vi "Trav_single_profile.vi"(3 "Simulate/Run":T1, 5 "Traverse line":T2 {"Row Duration (mins)" format="%#.1f"; "Row No" min=0; "Trace Gas Concentration (%)" min=0.0 format="%#.2f"; "Emission Rate (l/min)" format="%#.2f"; "Tunnel Speed" format="%#.2f"; "Start X" format="%#.2f"; "Start Y" format="%#.2f"; "Start Z" format="%#.2f"; "End X" format="%#.2f"; "End Y" format="%#.2f"; "End Z" format="%#.2f"; "Averaging time (min)" min=0.0 format="%#.1f"}) -> (0 "Error Messages":string, 1 "Status":T5, 2 "Traverse line Out":T2 {"Row Duration (mins)" format="%#.1f"; "Row No" min=0; "Trace Gas Concentration (%)" min=0.0 format="%#.2f"; "Emission Rate (l/min)" format="%#.2f"; "Tunnel Speed" format="%#.2f"; "Start X" format="%#.2f"; "Start Y" format="%#.2f"; "Start Z" format="%#.2f"; "End X" format="%#.2f"; "End Y" format="%#.2f"; "End Z" format="%#.2f"; "Averaging time (min)" min=0.0 format="%#.1f"})   [LabVIEW 2010]
uses:
  Gen Trav/Multi_Run_Status.ctl
  Gen Trav/Traverse_cluster.ctl
  Gen Trav/Spacing.ctl
  Controls/Multi_run_mode.ctl
  Controls/User_Specific_mode.ctl
  Controls/Save_Data.ctl
  Controls/Setup.ctl
  ADAM Client/Sub VIs/ADAM Controls/Traverse_Level_State.ctl
  Controls/Overhead.ctl
  Globals/Trav_pos_global.vi
  Globals/Meas_global.vi
panel:
  out "Pause message":string
  in  "Pause":bool
  out "Current position":dbl[](array[numeric]) format="%.2f"
  in  "stop":bool
  in  "Array of Positions":dbl[][](array[numeric]) format="%.2f"
  out "Abcissa copy":string="Y (mm)"
  out "Abcissa":string="Y (mm)"
  in  "Plot 1":i32[](listbox)=[1]
  out "Started Profile at:":string="16/9/98 12:33"
  out "Currently on point":i32=9
  out "U":cluster{dbl[], dbl[]}[](graph)
  out "% u'/U":cluster{dbl[], dbl[]}[](graph)
  # "X           Y            Z"
  # "Start"
  # "End"
  # "X           Y            Z"
  # "Start"
  # "End"
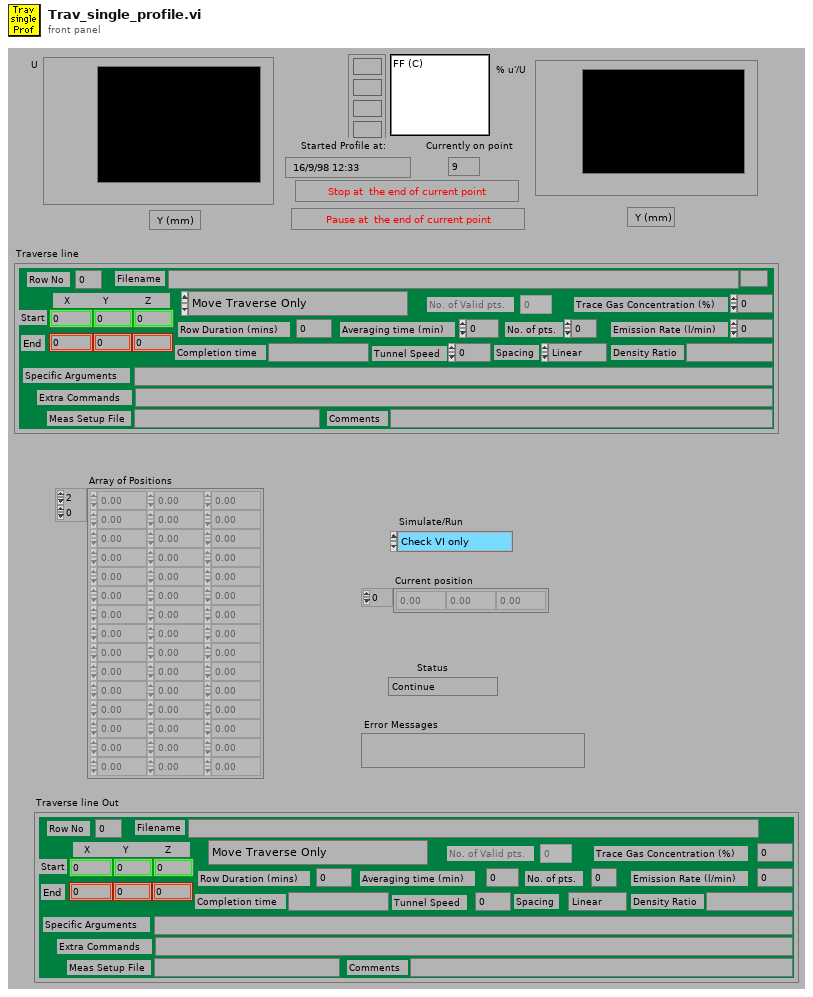
[diagram p1: front panel]
types:
  T1 = typedef "User_Specific_mode.ctl" = enum16{"Check VI only", "Run VI"}
  T2 = typedef "Traverse_cluster.ctl" = cluster{"Start X":dbl, "Start Y":dbl, "Start Z":dbl, "End X":dbl, "End Y":dbl, "End Z":dbl, "No. of pts.":i32, "Spacing":T3, "Filename":path, "Tunnel Speed":dbl, "Averaging time (min)":dbl, "Extra Commands":string, "Specific Arguments":string, "Emission Rate (l/min)":dbl, "Trace Gas Concentration (%)":dbl, "Density Ratio":string, "Comments":string, "Row No":i32, "Row Type Selector":T4, "Completion time":string, "Row Duration (mins)":dbl, "No. of Valid pts.":i32, "Meas Setup File":string}
  T3 = typedef "Spacing.ctl" = enum16{"Linear", "Log", "Gauss", "Specified", "N/A"}
  T4 = typedef "Multi_run_mode.ctl" = enum16{"Move Traverse Only", "Set Tunnel Speed Only", "Set Source Only", "Set Measurement Conditions", "Single Measurement", "Vertical Profile", "Lateral Profile", "Longitudinal Profile", "Explore Volume", "Multi-Axis Profile", "Auto Calibrate", "Meas Fast FID Bkgnd", "Check Beam Power", "Scanning Valve Measurement", "Run VI Named:", "Set ADAM Ch", "Wait (minutes)", "Send Message", "Synchronize With:", "Fall Back to this Row", "Turn Off Row Repeating", "Blank Row"}
  T5 = typedef "Multi_Run_Status.ctl" = enum16{"Continue", "Jump to Next Point", "Jump to Next Row", "Jump To Fall Back", "Terminate Run"}
  T6 = typedef "Save_Data.ctl" = enum16{"Save No Data", "Save Data"}
  T7 = typedef "Setup.ctl" = enum16{"Run Program", "Show Setup", "Save Current Setup", "Setup Front Panel"}
  T8 = typedef "Traverse_Level_State.ctl" = enum16{"Running", "Complete"}
  T9 = typedef "Overhead.ctl" = enum16{"Update total times", "Read Current Overhead", "Re Scale totals to 3 hrs", "Initialise totals to 3hr"}
  T10 = typedef "Status_Cluster.ctl" = cluster{"Status":T5, "Error Type":string, "Error Description":string}
  T11 = typedef "Velocity_cluster.ctl" = cluster{"Name":string, "U":dbl, "u^2":dbl, "u^3/(u^2)^(1.5)":dbl, "u^4/(u^2)^2 -3":dbl, "% u'/U":dbl, "Mean % Err":dbl, "u^4":dbl}
  T12 = typedef "Analysis_type_cluster.ctl" = cluster{"Analysis type":T13, "Indicies":i32[], "Name":string, "Inst Array":T14, "Info index":i32}
  T13 = typedef "Analysis_type_Enum.ctl" = enum16{"Slow Response", "Fast Response", "Weighted Fast Response", "Fast FID", "Weighted Fast FID", "Cross Wire", "Weighted Cross Wire", "Weighted LDA"}
  T14 = typedef "Instrument_Array.ctl" = enum16{"PWA", "LDA", "Analogue"}
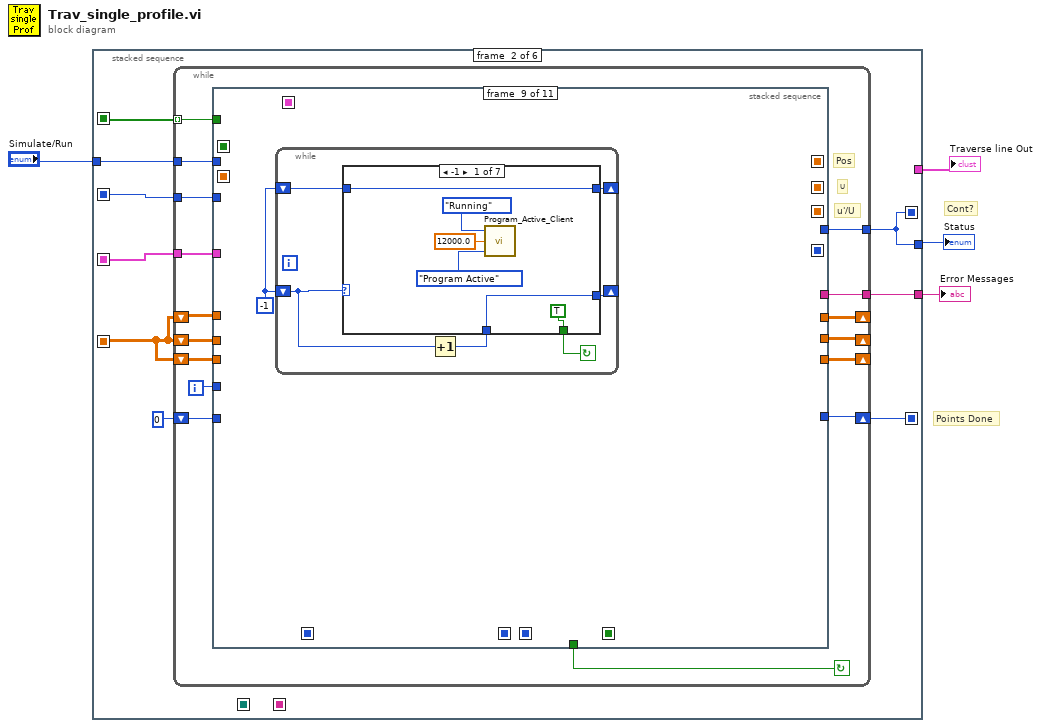
[diagram p0: block diagram]
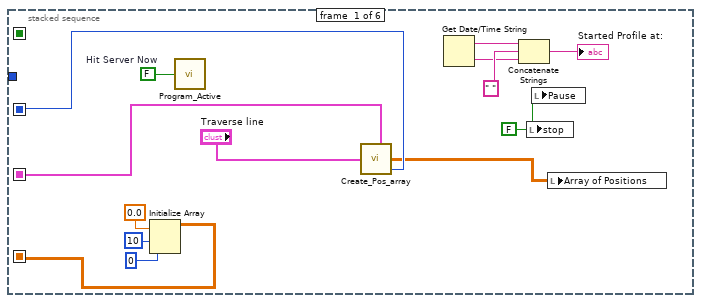
[diagram p2: hidden frame]
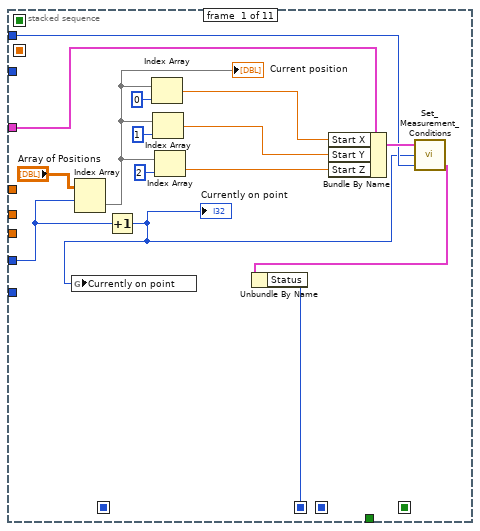
[diagram p3: hidden frame]
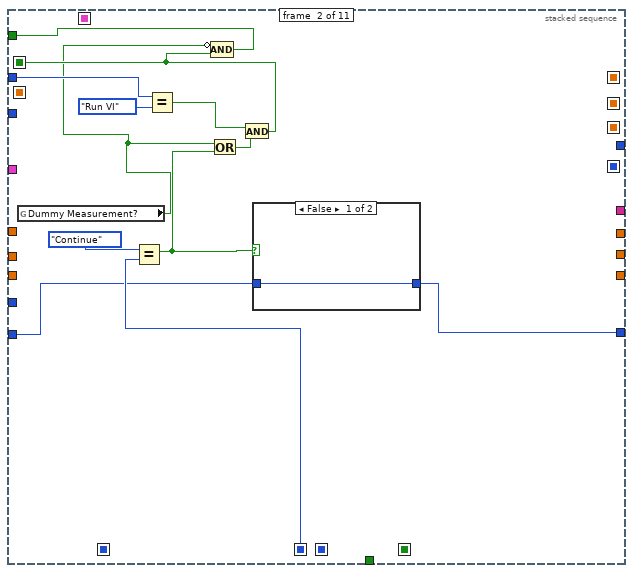
[diagram p4: hidden frame]
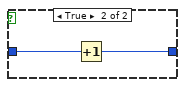
[diagram p5: hidden frame]
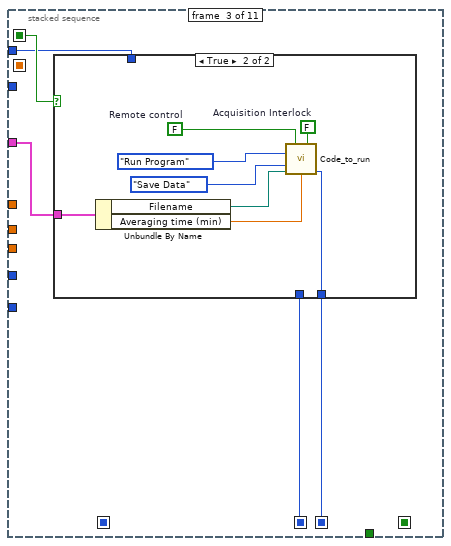
[diagram p6: hidden frame]
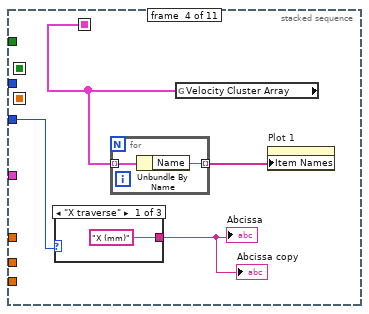
[diagram p8: hidden frame]
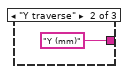
[diagram p9: hidden frame]
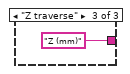
[diagram p10: hidden frame]
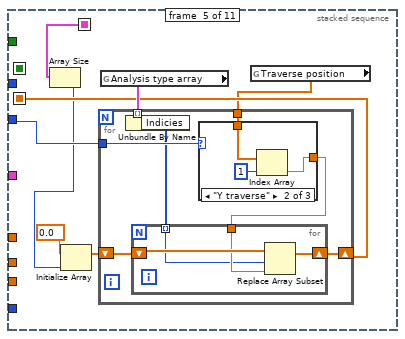
[diagram p11: hidden frame]
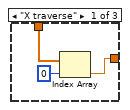
[diagram p12: hidden frame]
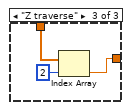
[diagram p13: hidden frame]
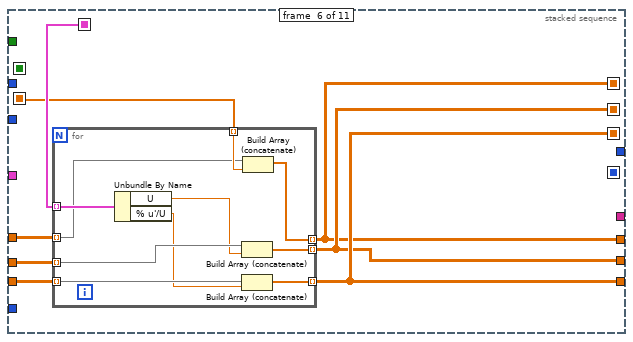
[diagram p14: hidden frame]
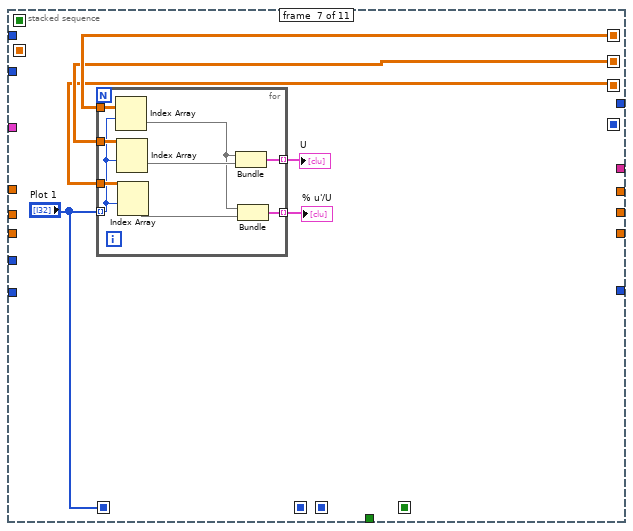
[diagram p15: hidden frame]
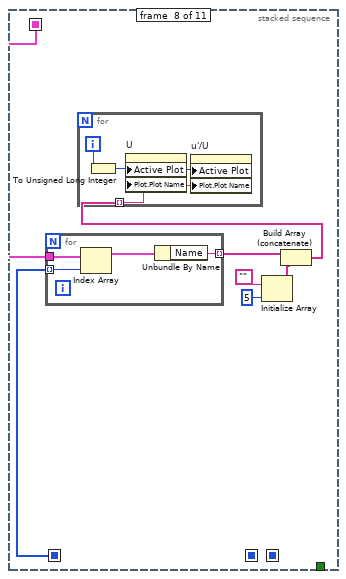
[diagram p16: hidden frame]
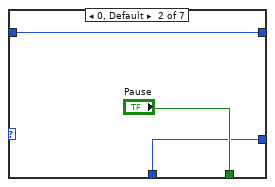
[diagram p17: hidden frame]
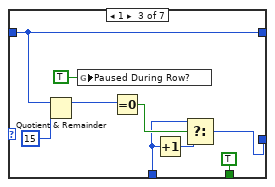
[diagram p18: hidden frame]
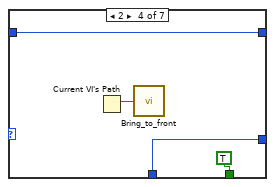
[diagram p19: hidden frame]
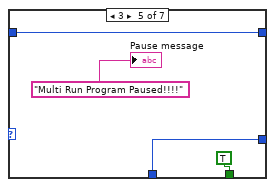
[diagram p20: hidden frame]
diagram:
  # "Points Done"
  # "Cont?"
  n1 = stacked-sequence {
    seq-local: [w11 _ _ _ _ _] -> [_ w26 _ _ _ _]
    seq-local: [w10 _ _ _ _ _] -> [_ w27 _ _ _ _]
    seq-local: [_ _ w276 _ _ _] -> [_ _ _ _ w300 _]
    seq-local: [_ _ _ w283 _ _] -> [_ _ _ _ w299 _]
    seq-local: [_ w25 _ _ _ _] -> [_ _ _ _ _ _]
    seq-local: [_ w23 _ _ _ _] -> [_ _ _ w280 w298 _]
    seq-local: [_ w21 _ _ _ _] -> [_ _ _ _ _ w305]
    seq-local: [w6 _ _ _ _ _] -> [_ w20 _ _ _ w307]
    tunnel: [_ w25 _ _ _ _] -> w2
    tunnel: [_ _ _ _ _ w317] -> w4
    tunnel: "Simulate/Run" -> [_ w24 _ _ _ w316]
    tunnel: [_ w19 _ _ _ _] -> w1
    frame #0 {
      w8 = FALSE ("stop")
      w9 = FALSE  # Hit Server Now
      n2 = Initialize Array(0.0, 10, 0) -> (w11:dbl[][])
      n3 = call "Program_Active.vi"("Hit Server Now"=w9) -> ()
      n4 = call "Create_Pos_array.vi"("Traverse line"="Traverse line") -> ("Traverse line Out"=w6:T2, "Array of Positions"=w5:dbl[][], "Axis Traversed"=w10:enum16{"X traverse", "Y traverse", "Z traverse"})  [unwired: 5 in, 1 out]
      n5 = Get Date/Time String() -> (date string=w17:string, time string=w16:string)  [unwired: 3 out]
      n6 = Concatenate Strings(w17, " ", w16) -> (→"Started Profile at:":string)
      n7 = local write "stop"(w8) -> ()
      n8 = local write "Pause"(w8) -> ()
      n9 = local write "Array of Positions"(w5) -> ()
    }
    frame #1 {
      n10 = while {
        shift-left: 0 -> [w30]
        shift-right: [w29] -> w21
        tunnel: [w31] -> w23 mode=indexing
        tunnel: w20 -> [w32]
        tunnel: w24 -> [w33]
        tunnel: [w34] -> w25
        shift-left: w26 -> [w37]
        shift-right: [w36] -> _
        tunnel: w27 -> [w38]
        shift-left: w26 -> [w40]
        shift-right: [w39] -> _
        shift-left: w26 -> [w42]
        shift-right: [w41] -> _
        tunnel: [w28] -> w19
        i -> [w43]
        stop <- w35 continue-if-true
        # "Pos"
        # "U"
        # "u'/U"
        n11 = stacked-sequence {
          seq-local: [_ _ _ _ w102 _ _ _ _ _ _] -> [_ _ _ _ _ w127 _ _ _ _ _]
          seq-local: [_ _ _ w91 _ _ _ _ _ _ _] -> [_ _ _ _ w101 w130 _ w158 _ _ _]
          seq-local: [_ _ _ _ _ w125 _ _ _ _ _] -> [_ _ _ _ _ _ w148 _ _ _ _]
          seq-local: [_ _ _ _ _ w128 _ _ _ _ _] -> [_ _ _ _ _ _ w147 _ _ _ _]
          seq-local: [_ _ _ _ _ w129 _ _ _ _ _] -> [_ _ _ _ _ _ w146 _ _ _ _]
          seq-local: [_ _ _ _ _ _ "Plot 1" _ _ _ _] -> [_ _ _ _ _ _ _ w164 _ _ _]
          seq-local: [_ _ w77 _ _ _ _ _ _ _ _] -> [_ _ _ _ _ _ _ _ _ w222 _]
          seq-local: [w48 _ _ _ _ _ _ _ _ _ _] -> [_ w68 w75 _ _ _ _ _ _ _ _]
          seq-local: [_ w61 _ _ _ _ _ _ _ _ _] -> [_ _ w76 _ _ _ _ _ _ _ _]
          seq-local: [_ _ _ _ _ _ _ _ _ w217 _] -> [_ _ _ _ _ _ _ _ _ _ w238]
          seq-local: [_ _ _ _ _ _ _ _ _ w216 _] -> [_ _ _ _ _ _ _ _ _ _ w232]
          tunnel: w43 -> [w45 _ _ _ _ _ _ _ _ w228 w235]
          tunnel: w42 -> [_ _ _ _ _ w132 _ _ _ _ _]
          tunnel: [_ _ _ _ _ w128 _ _ _ _ _] -> w41
          tunnel: w40 -> [_ _ _ _ _ w131 _ _ _ _ _]
          tunnel: [_ _ _ _ _ w129 _ _ _ _ _] -> w39
          tunnel: w38 -> [_ _ _ w89 w103 _ _ _ _ _ _]
          tunnel: w37 -> [_ _ _ _ _ w126 _ _ _ _ _]
          tunnel: [_ _ _ _ _ w125 _ _ _ _ _] -> w36
          tunnel: [_ _ _ _ _ _ _ _ _ w217 _] -> w35
          tunnel: w32 -> [w52 _ w78 _ _ _ _ _ _ _ w236]
          tunnel: [_ _ _ _ _ _ _ _ _ _ w234] -> w34
          tunnel: w33 -> [w50 w70 w74 _ _ _ _ _ _ _ w237]
          tunnel: [_ w60 _ _ _ _ _ _ _ _ _] -> w31
          tunnel: w30 -> [_ w65 _ _ _ _ _ _ _ _ _]
          tunnel: [_ w64 _ _ _ _ _ _ _ _ _] -> w29
          tunnel: [_ _ _ _ _ _ _ _ _ _ w233] -> w28
          frame #0 {
            n12 = Index Array(array="Array of Positions", index (row)=w45) -> (element=w44:dbl[])  [unwired: 1 in]
            "Current position" <- w44
            n13 = Increment(x=w45) -> (x+1=w47:i32)
            "Currently on point" <- w47
            n14 = global write "Trav_pos_global.vi" "Currently on point"(w47) -> ()
            n15 = Index Array(array=w44, index=0 ("Index")) -> (element=w55:dbl)
            n16 = Index Array(array=w44, index=1 ("Index")) -> (element=w54:dbl)
            n17 = Index Array(array=w44, index=2 ("Index")) -> (element=w53:dbl)
            n18 = Bundle By Name(cluster=w52, "Start X"=w55, "Start Y"=w54, "Start Z"=w53) -> (w51:T2)
            n19 = call "Set_Measurement_Conditions.vi"("Simulate/Run"=w50, "Currently on Point"=w47, "Traverse line"=w51) -> ("Status Cluster"=w49:T10)  [unwired: 2 out]
            n20 = Unbundle By Name(w49) -> ("Status"=w48:T5)
          }
          frame #1 {
            n21 = global read "Trav_pos_global.vi" "Dummy Measurement?"() -> (w59:bool)
            n22 = Equal?(x=Multi_Run_Status."Continue" ("Status"), y=w68) -> (x = y?=w63:bool)
            n23 = Equal?(x=w70, y=User_Specific_mode."Run VI" ("Simulate/Run")) -> (x = y?=w66:bool)
            n24 = Or(x=w59, y=w63) -> (x .or. y?=w62:bool)
            n25 = And(x=w66, y=w62) -> (x .and. y?=w61:bool)
            n26 = Compound Arithmetic op=AND(invert w59, w61) -> (w60:bool)
            n27 = case shown="False" w63 {
              tunnel: w65 -> [w71 w73]
              tunnel: [w71 w72] -> w64
              frame False {
              }
              frame True {
                n28 = Increment(x=w73) -> (x+1=w72:i32)
              }
            }
          }
          frame #2 {
            n29 = case shown="True" w76 {
              tunnel: w78 -> [_ w87]
              tunnel: [w79 w86] -> w77
              tunnel: w75 -> [w79 _]
              tunnel: w74 -> [_ _]
              frame False {
              }
              frame True {
                w82 = FALSE  # Acquisition Interlock
                w85 = FALSE  # Remote control
                n30 = Unbundle By Name(w87) -> ("Filename"=w83:path, "Averaging time (min)"=w84:dbl)
                n31 = call "Code_to_run.vi"("Acquisition Interlock"=w82, "setup"=Setup."Run Program", "Remote control"=w85, "File"=Save_Data."Save Data", "Results Filename"=w83, "Averaging time (min)"=w84) -> ("Status"=w86:T5)  [unwired: 5 in, 4 out]
              }
            }
          }
          frame #3 {
            n32 = case shown="\"X traverse\"" w89 {
              tunnel: ["X (mm)" "Y (mm)" "Z (mm)"] -> w88
              frame "X traverse" {
              }
              frame "Y traverse" {
              }
              frame "Z traverse" {
              }
            }
            "Abcissa" <- w88
            "Abcissa copy" <- w88
            n33 = global read "Meas_global.vi" "Velocity Cluster Array"() -> (w91:T11[])
            n34 = for {
              tunnel: w91 -> [w96] mode=indexing
              tunnel: [w95] -> w90 mode=indexing
              n35 = Unbundle By Name(w96) -> ("Name"=w95:string)
            }
            n36 = property on="Plot 1" class="LstBox (strict)"("Item Names"=w90) -> ()  [unwired: 2 in, 2 out]
          }
          frame #4 {
            n37 = Array Size(array=w101) -> (size(s)=w100:i32)
            n38 = Initialize Array(0.0, w100) -> (w98:dbl[])
            n39 = global read "Meas_global.vi" "Analysis type array"() -> (w104:T12[])
            n40 = global read "Trav_pos_global.vi" "Traverse position"() -> (w97:dbl[])
            n41 = for {
              shift-right: [w108] -> w102
              shift-left: w98 -> [w109]
              tunnel: w104 -> [w111] mode=indexing
              tunnel: w103 -> [w110]
              tunnel: w97 -> [w105]
              n42 = Unbundle By Name(w111) -> ("Indicies"=w106:i32[])
              n43 = case shown="\"Y traverse\"" w110 {
                tunnel: [w117 w120 w122] -> w107
                tunnel: w105 -> [w118 w119 w123]
                frame "X traverse" {
                  n44 = Index Array(array=w118, index=0) -> (element=w117:dbl)
                }
                frame "Y traverse" {
                  n45 = Index Array(array=w119, index=1) -> (element=w120:dbl)
                }
                frame "Z traverse" {
                  n46 = Index Array(array=w123, index=2) -> (element=w122:dbl)
                }
              }
              n47 = for {
                shift-right: [w114] -> w108
                shift-left: w109 -> [w115]
                tunnel: w107 -> [w113]
                tunnel: w106 -> [w112] mode=indexing
                n48 = Replace Array Subset(array=w115, new element=w113, index=w112) -> (w114:dbl[])
              }
            }
          }
          frame #5 {
            n49 = for {
              tunnel: w132 -> [w142] mode=indexing
              tunnel: [w140] -> w128 mode=indexing
              tunnel: w131 -> [w139] mode=indexing
              tunnel: [w137] -> w129 mode=indexing
              tunnel: w130 -> [w136] mode=indexing
              tunnel: w127 -> [w135] mode=indexing
              tunnel: w126 -> [w134] mode=indexing
              tunnel: [w133] -> w125 mode=indexing
              n50 = Unbundle By Name(w136) -> ("U"=w141:dbl, "% u'/U"=w138:dbl)
              n51 = Build Array (concatenate)(w142, w141) -> (w140:dbl[])
              n52 = Build Array (concatenate)(w139, w138) -> (w137:dbl[])
              n53 = Build Array (concatenate)(w134, w135) -> (w133:dbl[])
            }
          }
          frame #6 {
            n54 = for {
              tunnel: "Plot 1" -> [w149] mode=indexing
              tunnel: w148 -> [w157]
              tunnel: w147 -> [w156]
              tunnel: w146 -> [w155]
              tunnel: [w151] -> w145 mode=indexing
              tunnel: [w150] -> w144 mode=indexing
              n55 = Index Array(array=w157, index (row)=w149) -> (element=w153:dbl[])  [unwired: 1 in]
              n56 = Index Array(array=w156, index (row)=w149) -> (element=w154:dbl[])  [unwired: 1 in]
              n57 = Index Array(array=w155, index (row)=w149) -> (element=w152:dbl[])  [unwired: 1 in]
              n58 = Bundle(w153, w154) -> (w150:cluster{dbl[], dbl[]})  [unwired: 1 out]
              n59 = Bundle(w153, w152) -> (w151:cluster{dbl[], dbl[]})  [unwired: 1 out]
            }
            "U" <- w144
            "% u'/U" <- w145
          }
          frame #7 {
            n60 = for {
              tunnel: w164 -> [w168] mode=indexing
              tunnel: w158 -> [w166]
              tunnel: [w165] -> w161 mode=indexing
              n61 = Index Array(array=w166, index=w168) -> (element=w167:T11)
              n62 = Unbundle By Name(w167) -> ("Name"=w165:string)
            }
            n63 = Initialize Array("", 5) -> (w160:string[])
            n64 = Build Array (concatenate)(w161, w160) -> (w159:string[])
            n65 = for {
              tunnel: w159 -> [w169] mode=indexing
              i -> [w171]
              n66 = To Unsigned Long Integer(number=w171) -> (unsigned 32bit integer=w170:u32)
              n67 = property on="U" class="XYGraph (strict)"("Active Plot"=w170, "Plot.Plot Name"=w169) -> ()  [unwired: 2 in, 2 out]
              n68 = property on="u'/U" class="XYGraph (strict)"("Active Plot"=w170, "Plot.Plot Name"=w169) -> ()  [unwired: 2 in, 2 out]
            }
          }
          frame #8 {
            w172 = -1
            n69 = while {
              shift-left: w172 -> [w173]
              shift-right: [w174] -> _
              shift-left: w172 -> [w177]
              shift-right: [w178] -> _
              stop <- w175 continue-if-true
              n70 = Increment(x=w177) -> (x+1=w176:i32)
              n71 = case shown="-1" w177 {
                tunnel: [w183 w186 w190 w200 w203 w207 0] -> w178
                tunnel: w176 -> [w183 w186 w192 w200 w203 w207 _]
                tunnel: [TRUE ("Pause") "Pause" TRUE ("Pause") TRUE ("Pause") TRUE ("Pause") TRUE ("Pause") TRUE ("Pause")] -> w175
                tunnel: [w182 w185 w188 w197 w201 w205 w210] -> w174
                tunnel: w173 -> [w182 w185 w188 w197 w201 w205 w211]
                frame -1 {
                  n72 = call "Program_Active_Client.vi"("Mode"=enum16{"Program Active", "Traverse Level State"}."Program Active", "Time till next contact (Sec)"=12000.0, "Traverse level State"=Traverse_Level_State."Running") -> ()  [unwired: 3 out]
                }
                frame 0, Default {
                }
                frame 1 {
                  n73 = Quotient & Remainder(x=w188, y=15) -> (x-y*floor(x/y)=w194:i32)  [unwired: 1 out]
                  n74 = global write "Trav_pos_global.vi" "Paused During Row?"(TRUE ("Paused During Row?")) -> ()
                  n75 = Equal To 0?(x=w194) -> (x = 0?=w193:bool)
                  n76 = Increment(x=w192) -> (x+1=w191:i32)
                  n77 = Select(t=w192, s=w193, f=w191) -> (s? t:f=w190:i32)
                }
                frame 2 {
                  n78 = Current VI's Path() -> (path=w198:path)
                  n79 = call "Bring_to_front.vi"("path"=w198) -> ()
                }
                frame 3 {
                  "Pause message" <- "Multi Run Program Paused!!!!" ("Pause message")
                }
                frame 4 {
                  n80 = property on="Pause message" class="Str"("Visible"=TRUE) -> ()  [unwired: 2 in, 2 out]
                  n81 = Wait Until Next ms Multiple(millisecond multiple=u32 1500) -> ()  [unwired: 1 out]
                }
                frame 5 {
                  n82 = Increment(x=w211) -> (x+1=w210:i32)
                  n83 = property on="Pause message" class="Str"("Visible"=FALSE) -> ()  [unwired: 2 in, 2 out]
                  n84 = Wait Until Next ms Multiple(millisecond multiple=u32 1500) -> ()  [unwired: 1 out]
                }
              }
            }
          }
          frame #9 {
            n85 = Increment(x=w228) -> (x+1=w227:i32)
            n86 = local read "Array of Positions"() -> (w218:dbl[][])
            n87 = case shown="\"Jump to Next Point\"" w222 {
              tunnel: [TRUE TRUE FALSE] -> w225
              frame "Continue" {
              }
              frame "Jump to Next Point" {
              }
              frame "Jump to Next Row", Default {
              }
            }
            n88 = Array Size(array=w218) -> (size(s)=w221:i32[])
            n89 = Index Array(array=w221, index=0 ("Index")) -> (element=w219:i32)
            n90 = Less?(x=w227, y=w219) -> (x < y?=w226:bool)
            n91 = Compound Arithmetic op=AND(w225, invert "stop", w226) -> (w217:bool)
            n92 = Select(t=Multi_Run_Status."Terminate Run" ("Status"), s="stop", f=w222) -> (s? t:f=w216:T5)
          }
          frame #10 {
            n93 = case shown="True" w238 {
              tunnel: w237 -> [_ w247]
              tunnel: w236 -> [_ w246]
              tunnel: w235 -> [_ w245]
              tunnel: [w240 w242] -> w234
              tunnel: ["" w241] -> w233
              tunnel: w232 -> [w240 _]
              frame False {
              }
              frame True {
                n94 = case shown="\"Check VI only\"" w247 {
                  tunnel: w246 -> [w263 _]
                  tunnel: w245 -> [w258 _]
                  tunnel: [w248 timestamp(0 s since 1904-01-01)] -> w244
                  frame "Check VI only" {
                    n95 = Increment(x=w258) -> (x+1=w256:i32)
                    n96 = Unbundle By Name(w263) -> ("Averaging time (min)"=w260:dbl)
                    n97 = global read "Trav_pos_global.vi" "Simulation Time"() -> (w250:timestamp)
                    n98 = To Double Precision Float(number=w250) -> (double precision float=w251:dbl)
                    n99 = Multiply(x=60.0, y=w260) -> (x*y=w259:dbl)
                    n100 = Add(x=w259, y=10.0 ("Scalable Time (Sec)")) -> (x+y=w257:dbl)
                    n101 = Multiply(x=w257, y=w256) -> (x*y=w254:dbl)
                    n102 = call "Overhead_Factor.vi"("Mode"=Overhead."Read Current Overhead") -> ("Current Overhead Factor"=w255:dbl)  [unwired: 3 in]
                    n103 = Multiply(x=w255, y=w254) -> (x*y=w252:dbl)
                    n104 = Add(x=w251, y=w252) -> (x+y=w249:dbl)
                    n105 = To Time Stamp(1:w249) -> (0:w248:timestamp)
                  }
                  frame "Run VI" {
                  }
                }
                n106 = call "Run_FFID_Bkgnd.vi"("Simulated Time"=w244, "Run Now?"=FALSE, "Simulate/Run"=w247) -> ("Error Messages"=w241:string, "Status"=w242:T5)  [unwired: 1 out]
              }
            }
          }
        }
      }
    }
    frame #2 {
      n107 = global read "Meas_global.vi" "Start Time of experiment"() -> (w266:dbl)
      n108 = global read "Meas_global.vi" "Raw data file"() -> (w278:path)
      n109 = Strip Path(path=w278) -> (stripped path=w277:path)  [unwired: 1 out]
      n110 = call "Sec_to_date_filename.vi"("seconds"=w266) -> ("Day"=w268:string, "Time"=w269:string)  [unwired: 2 out]
      n111 = Format Into String(format string="Cmd_%s_%s.xls", w268, w269) -> (resulting string=w271:string)  [unwired: 2 in, 1 out]
      n112 = call "Fast_string_Replace.vi"("Replace match with:"="-", "Input String"=w271, "regular expression"=":") -> ("Output String"=w274:string)  [unwired: 2 out]
      n113 = call "Fast_string_Replace.vi"("Replace match with:"="", "Input String"=w274, "regular expression"=" ") -> ("Output String"=w265:string)  [unwired: 2 out]
      n114 = Build Path(base path=w277, name or relative path=w265) -> (appended path=w276:path)
    }
    frame #3 {
      w289 = "\t"
      n115 = local read "Array of Positions"() -> (w282:dbl[][])
      n116 = Number To Fractional String(number=w282, precision (6)=i16 2) -> (F-format string=w281:string[][])  [unwired: 2 out]
      n117 = for {
        tunnel: w281 -> [w294] mode=indexing
        tunnel: w280 -> [w293] mode=indexing
        tunnel: [w291] -> w279 mode=indexing
        n118 = case shown="False" w293 {
          tunnel: ["Unobtainable Position" ""] -> w292
          frame False {
          }
          frame True {
          }
        }
        n119 = Build Array (concatenate)(w294, w292) -> (w291:string[])
      }
      n120 = Concatenate Strings("X", w289, "Y", w289, "Z") -> (w284:string)
      n121 = call "2D_array_to_string.vi"("2D data array"=w279, "Column titles  (separated by tabs)"=w284, "Array title"="Requested positions") -> ("Output string"=w283:string)
    }
    frame #4 {
      n122 = Or Array Elements(Boolean array=w298) -> (logical OR=w297:bool)
      n123 = case shown="True" w297 {
        tunnel: w300 -> [_ w303]
        tunnel: w299 -> [_ w301]
        frame False {
        }
        frame True {
          w302 = FALSE  # Lock File
          w304 = TRUE  # append to file? (new file:F)
          n124 = call "Write_Characters_To_File.vi"("file path (dialog if empty)"=w303, "character string"=w301, "append to file? (new file:F)"=w304, "Lock File"=w302) -> ()  [unwired: 1 in, 4 out]
        }
      }
    }
    frame #5 {
      n125 = local read "Array of Positions"() -> (w309:dbl[][])
      n126 = Array Size(array=w309) -> (size(s)=w311:i32[])
      n127 = Index Array(array=w311, index=0 ("Index")) -> (element=w308:i32)
      n128 = Bundle By Name(cluster=w307, "No. of Valid pts."=w305) -> (w306:T2)
      n129 = Not Equal?(x=w308, y=w305) -> (x != y?=w314:bool)
      n130 = Equal?(x=User_Specific_mode."Run VI" ("Simulate/Run"), y=w316) -> (x = y?=w313:bool)
      n131 = And(x=w313, y=w314) -> (x .and. y?=w312:bool)
      n132 = case shown="True" w312 {
        tunnel: w306 -> [w318 w330]
        tunnel: [w318 w329] -> w317
        tunnel: w305 -> [_ w328]
        frame False {
        }
        frame True {
          w319 = " !!Program added comments"
          n133 = Unbundle By Name(w330) -> ("Comments"=w320:string)
          n134 = Equal To 0?(x=w328) -> (x = 0?=w327:bool)
          n135 = Match Pattern(string=w320, regular expression=w319) -> (match substring=w322:string)  [unwired: 4 out]
          n136 = Select(t=" !!(Row Skipped)", s=w327, f=" !!(Row Partially Skipped)") -> (s? t:f=w323:string)
          n137 = Empty String/Path?(string/path=w322) -> (empty?=w321:bool)
          n138 = case shown="True" w321 {
            tunnel: [w333 w337] -> w324
            tunnel: w323 -> [w332 w336]
            tunnel: w319 -> [_ w335]
            tunnel: w320 -> [w331 w334]
            frame False {
              n139 = Concatenate Strings(w331, w332) -> (w333:string)
            }
            frame True {
              n140 = Concatenate Strings(w334, w335, w336) -> (w337:string)
            }
          }
          n141 = Bundle By Name(cluster=w330, "Comments"=w324) -> (w329:T2)
        }
      }
    }
  }
  "Status" <- w2
  "Traverse line Out" <- w4
  "Error Messages" <- w1
